vi "receiveData.vi"(8 "error in (no error)":errorcluster, 11 "Controller.LV in":refnum<class "Controller.LV.lvclass">) -> (0 "error out":errorcluster, 3 "Controller.LV out":refnum<class "Controller.LV.lvclass">)   [LabVIEW 2019, in "Controller.LV.lvclass"]
uses:
  Controller.LV.lvclass
  Controller.LV.lvclass/Controller.LV.ctl
  drivers/Class/Controller/Controller.lvclass
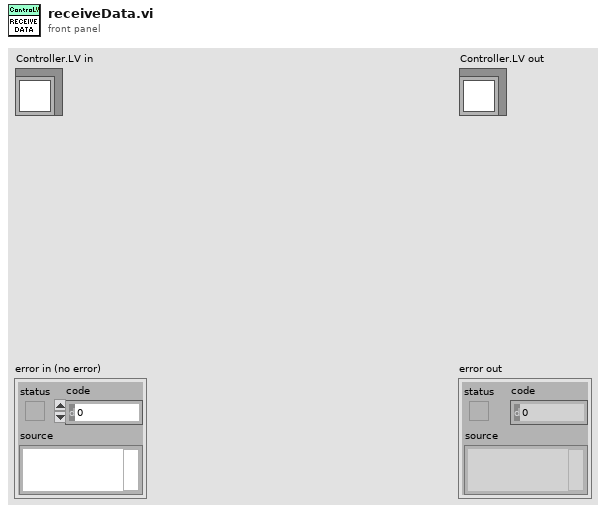
[diagram p1: front panel]
types:
  T1 = cluster{"SRNO":dbl, "SOFT":dbl, "STAT":dbl, "FREQ":dbl, "OFRQ":dbl, "CURR":dbl, "SYNC":dbl, "Encoder Position [enc. units]":dbl, "Desired Position [enc. units]":dbl, "TIME":dbl}
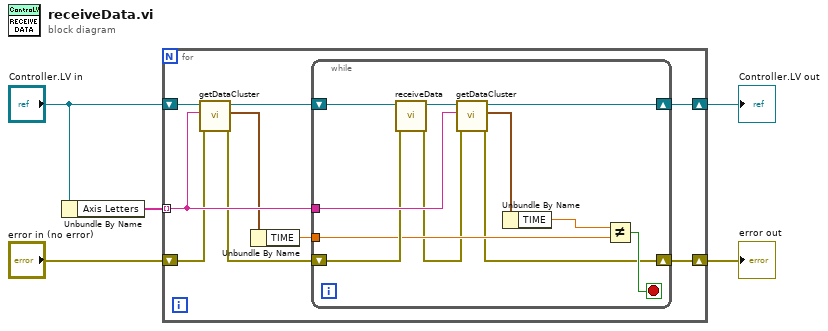
[diagram p0: block diagram]
diagram:
  n1 = Unbundle By Name("Controller.LV in") -> ("Axis Letters"=w1:string[])
  n2 = for {
    shift-right: [w14] -> w5
    shift-left: "error in (no error)" -> [w9]
    shift-right: [w13] -> w3
    shift-left: "Controller.LV in" -> [w11]
    tunnel: w1 -> [w12] mode=indexing
    n3 = call-dynamic "getDataCluster.vi"("error in (no error)"=w9, "Axis Letter"=w12, "Controller in"=w11) -> ("error out"=w8:errorcluster, "Information"=w7:T1, "Controller out"=w10:refnum<class "Controller.LV.lvclass">)  [unwired: 6 in]
    n4 = Unbundle By Name(w7) -> ("TIME"=w6:dbl)
    n5 = while {
      tunnel: w12 -> [w22]
      shift-right: [w23] -> w13
      shift-left: w10 -> [w21]
      shift-right: [w15] -> w14
      shift-left: w8 -> [w20]
      tunnel: w6 -> [w18]
      stop <- w17 stop-if-true
      n6 = call-parent "receiveData.vi"("error in (no error)"=w20, "Controller in"=w21) -> ("error out"=w16:errorcluster, "Controller out"=w24:refnum<class "Controller.LV.lvclass">)  [unwired: 8 in]
      n7 = call-dynamic "getDataCluster.vi"("error in (no error)"=w16, "Axis Letter"=w22, "Controller in"=w24) -> ("error out"=w15:errorcluster, "Information"=w25:T1, "Controller out"=w23:refnum<class "Controller.LV.lvclass">)  [unwired: 6 in]
      n8 = Unbundle By Name(w25) -> ("TIME"=w19:dbl)
      n9 = Not Equal?(x=w19, y=w18) -> (x != y?=w17:bool)
    }
  }
  "error out" <- w5
  "Controller.LV out" <- w3
